vi "ECUMC 2 Selection Dialog.vi"(8 "error in (no error)":errorcluster, 9 "NIVS.System Definition Root":refnum<k24>, 11 "Links in":T1) -> (0 "error out":errorcluster, 3 "Links out":T1)   [LabVIEW 2011]
doc: "Use this template to create a dialog box with event handling."
uses:
  NationalInstruments.VeriStand.SystemStorage
  Controls/Control Links.ctl
  Controls/ECUMC Item.ctl
  <vilib>/ECUMC/NIVS/Support Files.llb/Item Type.ctl
  <vilib>/ECUMC/NIVS/Support Files.llb/XCP and CCP Master Custom Device.lvlib
panel:
  in  "YMeas":bool
  in  "XMeas":bool
  in  "YChar":bool
  in  "XChar":bool
  out "Y Value":string
  out "X Index":string
  in  "Cancel":bool
  in  "Ok":bool
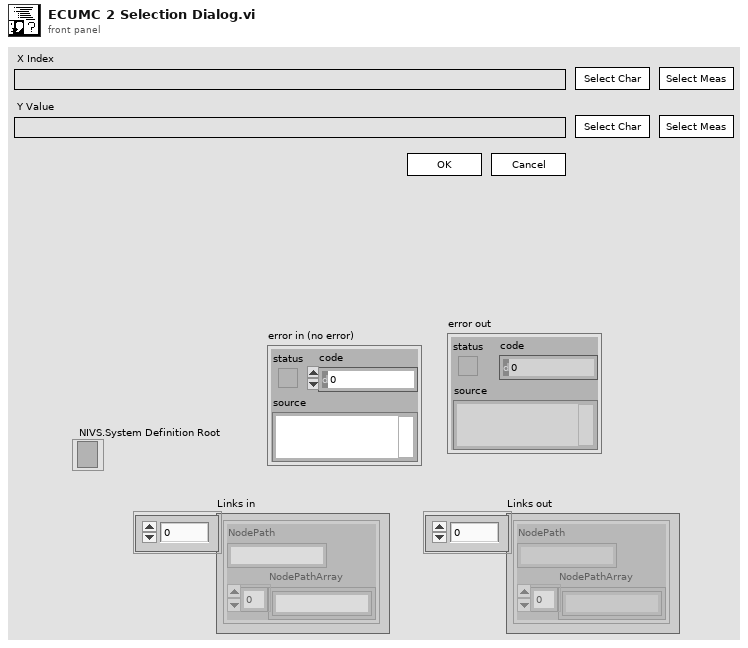
[diagram p1: front panel]
types:
  T1 = typedef "Control Links.ctl" = T2[]
  T2 = typedef "ECUMC Item.ctl" = cluster{"NodePath":string, "NodePathArray":string[]}
  T3 = typedef "XCP and CCP Master Custom Device.lvlib/Item Type.ctl" = enum16{"Scalar Characteristic", "Curve Characteristic", "Field Characteristic", "Measurement"}
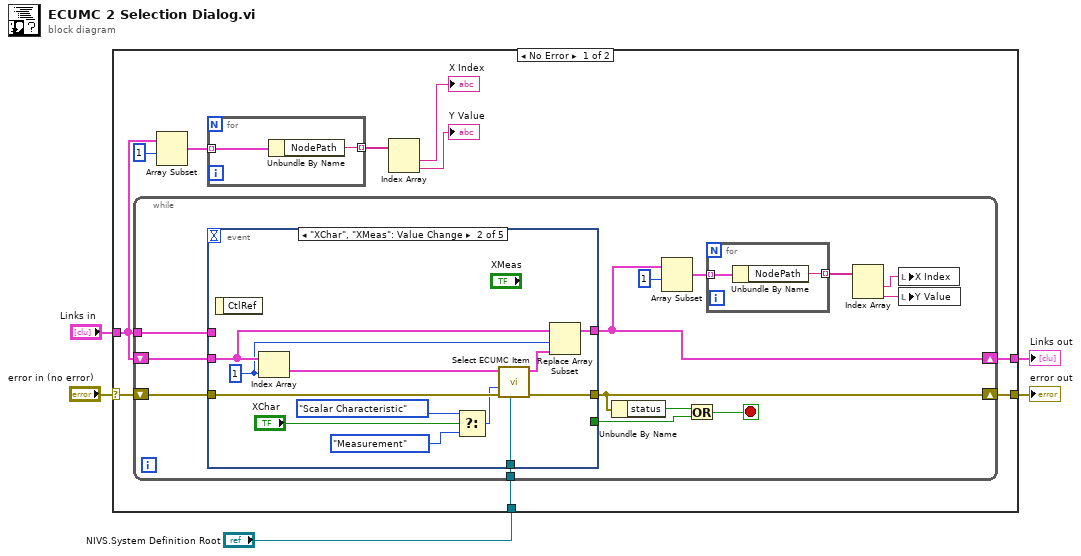
[diagram p0: block diagram]
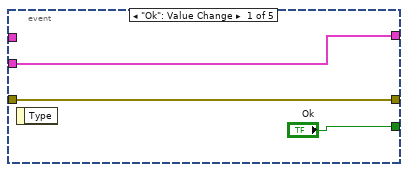
[diagram p2: hidden frame]
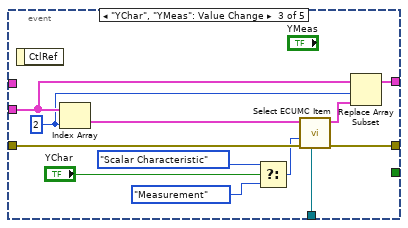
[diagram p3: hidden frame]
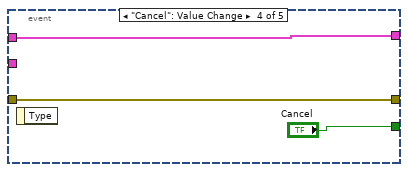
[diagram p4: hidden frame]
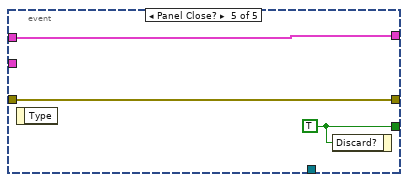
[diagram p5: hidden frame]
diagram:
  n1 = case shown="No Error" "error in (no error)" {
    selector: "error in (no error)" -> [w15 w68]
    tunnel: [w14 w68] -> w4
    tunnel: [w8 w67] -> w3
    tunnel: "Links in" -> [w7 w67]
    tunnel: "NIVS.System Definition Root" -> [w6 _]
    frame No Error {
      n2 = while {
        shift-right: [w27] -> w14
        shift-left: w15 -> [w28]
        shift-right: [w20] -> w8
        shift-left: w7 -> [w26]
        tunnel: w7 -> [w25]
        tunnel: w6 -> [w24]
        stop <- w30 stop-if-true
        n3 = event shown="[1] \"XChar\", \"XMeas\": Value Change" {
          selector: _ -> [_ _ _ _ _]
          dyn-events: _ -> [_ _ _ _ _]
          timeout: _ -> [_ _ _ _ _]
          tunnel: ["Ok" _ _ "Cancel" w66] -> w31
          tunnel: [w35 w47 w59 w61 w65] -> w27
          tunnel: w28 -> [w35 w48 w60 w61 w65]
          tunnel: w26 -> [w34 w44 w56 _ _]
          tunnel: [w34 w43 w55 w62 w64] -> w20
          tunnel: w25 -> [_ _ _ w62 w64]
          tunnel: w24 -> [_ w46 w58 _ _]
          event "Ok": Value Change {
            n4 = event-data() -> ()  [unwired: 1 in, 1 out]
          }
          event "XChar", "XMeas": Value Change {
            w41 = 1 ("index")
            n5 = event-data() -> ()  [unwired: 1 in, 1 out]
            n6 = Index Array(array=w44, index=w41) -> (element=w45:T2)
            n7 = Select(t=Item_Type."Scalar Characteristic" ("Item Type"), s="XChar", f=Item_Type."Measurement" ("Item Type")) -> (s? t:f=w37:T3)
            n8 = call "Select ECUMC Item.vi"("NIVS.System Definition Root"=w46, "error in (no error)"=w48, "Item Type"=w37, "Link In"=w45) -> ("error out"=w47:errorcluster, "Link Out"=w42:T2)  [unwired: 5 in, 1 out]
            n9 = Replace Array Subset(array=w44, new element=w42, index=w41) -> (w43:T1)
          }
          event "YChar", "YMeas": Value Change {
            w53 = 2 ("index")
            n10 = event-data() -> ()  [unwired: 1 in, 1 out]
            n11 = Index Array(array=w56, index=w53) -> (element=w57:T2)
            n12 = Select(t=Item_Type."Scalar Characteristic" ("Item Type"), s="YChar", f=Item_Type."Measurement" ("Item Type")) -> (s? t:f=w50:T3)
            n13 = call "Select ECUMC Item.vi"("NIVS.System Definition Root"=w58, "error in (no error)"=w60, "Item Type"=w50, "Link In"=w57) -> ("error out"=w59:errorcluster, "Link Out"=w54:T2)  [unwired: 5 in, 1 out]
            n14 = Replace Array Subset(array=w56, new element=w54, index=w53) -> (w55:T1)
          }
          event "Cancel": Value Change {
            n15 = event-data() -> ()  [unwired: 1 in, 1 out]
          }
          event Panel Close? {
            w66 = TRUE ("Cancel")
            n16 = event-data() -> ()  [unwired: 1 in, 1 out]
            n17 = event-data("Discard?"=w66) -> ()  [unwired: 1 in, 1 out]
          }
        }
        n18 = Unbundle By Name(w27) -> ("status"=w29:bool)
        n19 = Array Subset(array=w20, index=1) -> (w22:T1)  [unwired: 1 in]
        n20 = Or(x=w29, y=w31) -> (x .or. y?=w30:bool)
        n21 = for {
          tunnel: w22 -> [w33] mode=indexing
          tunnel: [w32] -> w23 mode=indexing
          n22 = Unbundle By Name(w33) -> ("NodePath"=w32:string)
        }
        n23 = Index Array(array=w23) -> (element #1=w19:string, element #2=w18:string)  [unwired: 2 in]
        n24 = local write "X Index"(w19) -> ()
        n25 = local write "Y Value"(w18) -> ()
      }
      n26 = Array Subset(array=w7, index=1) -> (w12:T1)  [unwired: 1 in]
      n27 = for {
        tunnel: w12 -> [w17] mode=indexing
        tunnel: [w16] -> w11 mode=indexing
        n28 = Unbundle By Name(w17) -> ("NodePath"=w16:string)
      }
      n29 = Index Array(array=w11) -> (element #1=→"X Index":string, element #2=→"Y Value":string)  [unwired: 2 in]
    }
    frame Error {
    }
  }
  "error out" <- w4
  "Links out" <- w3
